vi "Close Module.vi"(8 "error in (no error)":errorcluster, 9 "Wait for stop?":bool, 11 "Module Admin in":refnum<class "Delacor_lib_QMH_Cloneable Module Admin.lvclass">) -> (0 "error out":errorcluster, 1 "External Launch":bool, 3 "Module Admin out":refnum<class "Delacor_lib_QMH_Cloneable Module Admin.lvclass">)   [LabVIEW 2022 SP3, in "hse-db.lvlib" / "DB_CONNECTOR.lvlib"]
doc: "Destroy the Broadcast Events and Request Events (if this was the first instance). Reset flags stored in Module Admin class.\n____\nHAMPEL SOFTWARE ENGINEERING v1.4.0 (2023-12-19 09:52)"
uses:
  DB_CONNECTOR.lvlib
  <vilib>/Delacor/Delacor QMH/Libraries/Cloneable Module Admin_class/Delacor_lib_QMH_Cloneable Module Admin.lvclass
  C:/Program Files/National Instruments/LabVIEW 2022/vi.lib/Delacor/Delacor QMH/Libraries/Module Admin_class/Delacor_lib_QMH_Module Admin.lvclass
  Stop Argument--cluster.ctl
  <vilib>/Delacor/Delacor QMH/Libraries/Cloneable Module Admin_class/Delacor_lib_QMH_Cloneable Module Admin.lvclass/Delacor_lib_QMH_Cloneable Module Admin.ctl
  <vilib>/Delacor/Delacor QMH/Libraries/Module Admin_class/Delacor_lib_QMH_Module Admin.lvclass/Delacor_lib_QMH_Module Admin.ctl
  <vilib>/Delacor/Delacor QMH/Libraries/Cloneable Module Admin_class/Delacor_lib_QMH_Get First.vi
  <vilib>/Delacor/Delacor QMH/Libraries/Cloneable Module Admin_class/Delacor_lib_QMH_Get Module ID.vi
  <vilib>/Delacor/Delacor QMH/Libraries/Module Admin_class/Delacor_lib_QMH_Get External Launch.vi
  Clone Registration/Clone Registration.lvlib
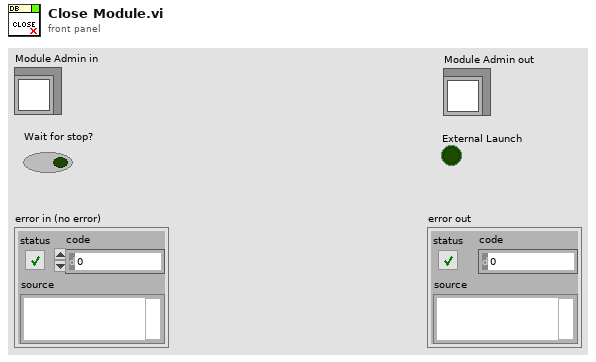
[diagram p1: front panel]
types:
  T1 = typedef "hse-db.lvlib/DB_CONNECTOR.lvlib/Stop Argument--cluster.ctl" = cluster{"Origin":string, "Module ID":i32, "Exit via Stop Module Req?":bool, "Wait for Module to stop?":bool}
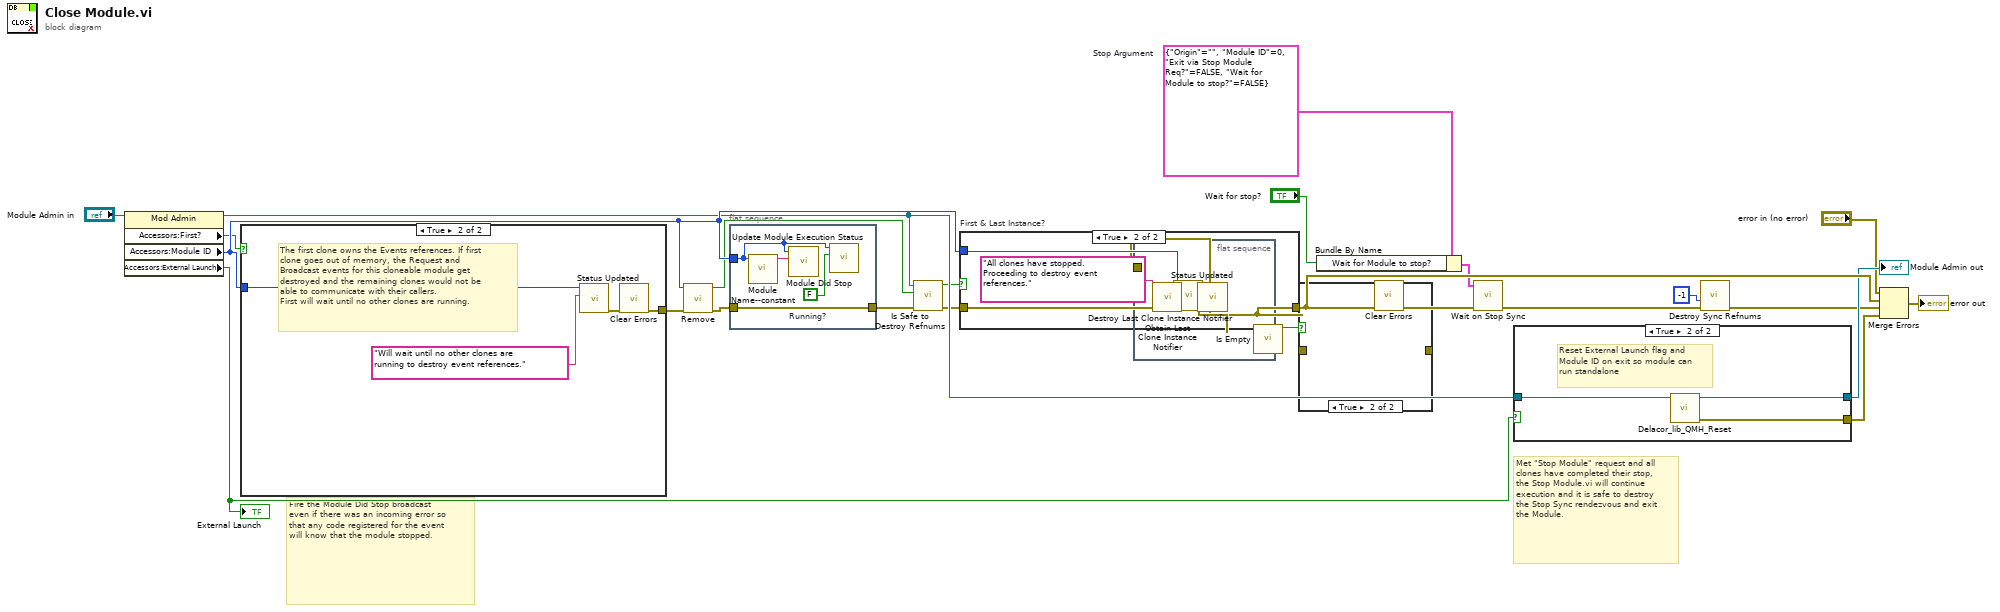
[diagram p0: block diagram]
diagram:
  w3 = T1 {"Origin"="", "Module ID"=0, "Exit via Stop Module Req?"=FALSE, "Wait for Module to stop?"=FALSE}  # Stop Argument
  # "Fire the Module Did Stop broadcast even if there was an incoming error so that any code registered for the event will know that the module stopped."
  # "Met \"Stop Module\" request and all clones have completed their stop, the Stop Module.vi will continue execution and it is safe to destroy the Stop Sync rendezvous and exit the Module."
  n1 = property class="Mod Admin"(reference="Module Admin in") -> (reference out=w18:refnum<class "Delacor_lib_QMH_Cloneable Module Admin.lvclass">, "Accessors:First?"=w9:bool, "Accessors:Module ID"=w22:i32, "Accessors:External Launch"=w8:bool)  [unwired: 1 in, 1 out]
  "External Launch" <- w8
  n2 = case shown="True" w9 {
    tunnel: w22 -> [_ w26]
    tunnel: [_ w24] -> w23
    frame False {
    }
    frame True {
      # "The first clone owns the Events references. If first clone goes out of memory, the Request and Broadcast events for this cloneable module get destroyed and the remaining clones would not be able to communicate with their callers.\nFirst will wait until no other clones are running."
      n3 = call "Status Updated.vi"("Status"="Will wait until no other clones are running to destroy event references." ("format string"), "Module ID"=w26) -> ("error out"=w25:errorcluster)  [unwired: 9 in]
      n4 = call <vilib>:"Clear Errors.vi"("error in (no error)"=w25) -> ("error out"=w24:errorcluster)  [unwired: 5 in, 1 out]
    }
  }
  n5 = call "Remove.vi"("error in (no error)"=w23, "Module ID"=w22) -> ("error out"=w19:errorcluster, "empty"=w6:bool)  [unwired: 7 in, 1 out]
  n6 = flat-sequence {
    tunnel: w19 -> [w31]
    tunnel: [w31] -> w5
    tunnel: w22 -> [w29]
    frame #0 {
      w28 = FALSE  # Running?
      n7 = call "Module Name--constant.vi"("Module ID"=w29) -> ("Module Name"=w30:string)  [unwired: 10 in]
      n8 = call "Module Did Stop.vi"("Origin"=w30, "Module ID"=w29) -> ()  [unwired: 9 in, 1 out]
      n9 = call "Update Module Execution Status.vi"("Running?"=w28, "Module ID"=w29) -> ()  [unwired: 9 in, 1 out]
    }
  }
  n10 = call "Is Safe to Destroy Refnums.vi"("error in (no error)"=w5, "empty"=w6, "Module Admin"=w18) -> ("error out"=w15:errorcluster, "Destroy Broadcast & Request Event Refs?"=w16:bool)  [unwired: 7 in]
  n11 = case "First & Last Instance?" shown="True" w16 {
    tunnel: w15 -> [w32 w39]
    tunnel: [w32 w35] -> w21
    tunnel: w22 -> [_ w38]
    frame False {
    }
    frame True {
      n12 = flat-sequence {
        tunnel: w35 -> [_]
        frame #0 {
          n13 = call "Obtain Last Clone Instance Notifier.vi"() -> ("Last Instance Notifier"=w44:refnum<notifier>)  [unwired: 10 in, 1 out]
          n14 = call "Destroy Last Clone Instance Notifier.vi"("Last Instance Notifier"=w44) -> ()  [unwired: 11 in]
        }
      }
      n15 = call "Status Updated.vi"("error in (no error)"=w39, "Status"="All clones have stopped. Proceeding to destroy event references.", "Module ID"=w38) -> ("error out"=w36:errorcluster)  [unwired: 8 in]
      n16 = call "Is Empty.vi"("error in (no error)"=w36) -> ("error out"=w33:errorcluster, "Empty?"=w34:bool)  [unwired: 9 in]
      n17 = case shown="True" w34 {
        tunnel: w33 -> [w40 w43]
        tunnel: [w40 w41] -> w35
        frame False {
        }
        frame True {
          n18 = call "Destroy Broadcast Events.vi"("error in (no error)"=w43) -> ("error out"=w42:errorcluster)  [unwired: 10 in]
          n19 = call "Destroy Request Events.vi"("error in (no error)"=w42) -> ("error out"=w41:errorcluster)  [unwired: 10 in]
        }
      }
    }
  }
  n20 = Bundle By Name(cluster=w3, "Wait for Module to stop?"="Wait for stop?") -> (w2:T1)
  n21 = call <vilib>:"Clear Errors.vi"("error in (no error)"=w21) -> ("error out"=w11:errorcluster)  [unwired: 5 in, 1 out]
  n22 = call "Wait on Stop Sync.vi"("error in"=w11, "Stop Argument"=w2) -> ("error out"=w4:errorcluster)  [unwired: 9 in]
  n23 = case shown="True" w8 {
    tunnel: w18 -> [w45 w48]
    tunnel: [w45 w47] -> w14
    tunnel: [_ w46] -> w20
    frame False {
    }
    frame True {
      # "Reset External Launch flag and Module ID on exit so module can run standalone"
      n24 = call-dynamic "Delacor_lib_QMH_Reset.vi"("Mod Admin in"=w48) -> ("error out"=w46:errorcluster, "Mod Admin out"=w47:refnum<class "Delacor_lib_QMH_Cloneable Module Admin.lvclass">)  [unwired: 9 in]
    }
  }
  "Module Admin out" <- w14
  n25 = call "Destroy Sync Refnums.vi"("error in (no error)"=w4, "Module ID"=-1) -> ("error out"=w13:errorcluster)  [unwired: 9 in]
  n26 = Merge Errors("error in (no error)", w21, w13, w20) -> (→"error out":errorcluster)
